vi "AfficherCommande.vi"() -> (0 "Result Set":string[][](table), 1 "Column Names":string[](array[string]))   [LabVIEW 2024]
uses:
  <vilib>/drjdpowell/SQLite Library/SQL Statement/SQL Statement.lvclass/SQL Statement.ctl
  <vilib>/drjdpowell/SQLite Library/SQL Connection/Open (string).vi
  <vilib>/drjdpowell/SQLite Library/SQL Connection/Execute SQL.vi
  <vilib>/drjdpowell/SQLite Library/SQL Statement/Error Message.vi
  <vilib>/drjdpowell/SQLite Library/SQL Connection/Connection.lvclass
  <vilib>/drjdpowell/SQLite Library/SQLite.lvlib
panel:
  # "Liste des commandes"
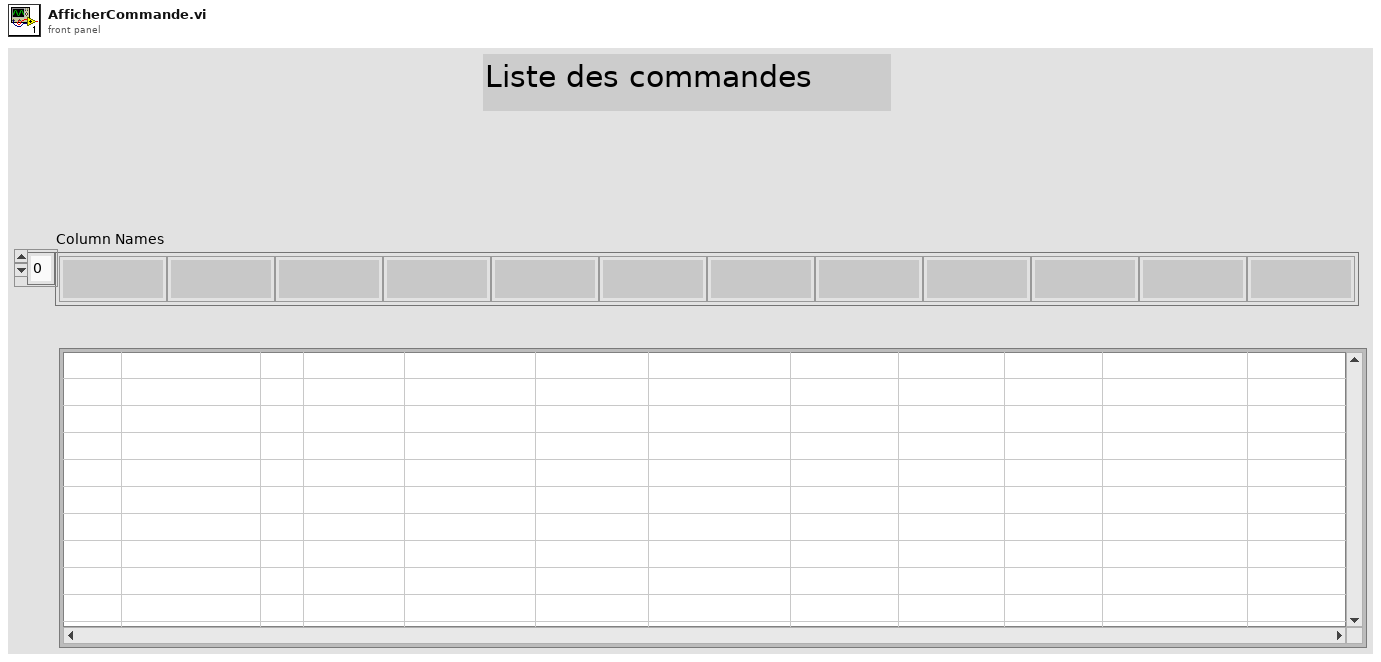
[diagram p1: front panel]
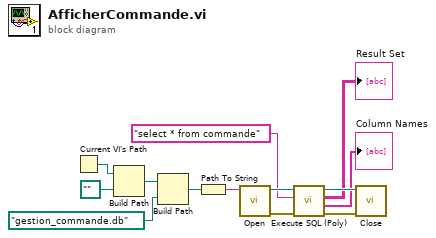
[diagram p0: block diagram]
diagram:
  n1 = Current VI's Path() -> (path=w13:path)
  n2 = Build Path(base path=w13, name or relative path=path "..") -> (appended path=w10:path)
  n3 = Build Path(base path=w10, name or relative path=path "gestion_commande.db" ("Filename")) -> (appended path=w9:path)
  n4 = Path To String(path=w9) -> (string=w1:string)
  n5 = call-poly <vilib>:"Open.vi"("db file"=w1) -> ("error out"=w7:errorcluster, "SQLite Connection"=w8:refnum<class "Connection.lvclass">)  [unwired: 9 in]
  n6 = call-poly <vilib>:"Execute SQL (Poly).vi"("error in (no error)"=w7, "SQL"="select * from commande", "SQLite Connection in"=w8) -> ("error out"=w6:errorcluster, "Column Names"=→"Column Names":string[], "Result Set"=→"Result Set":string[][], "SQLite Connection"=w5:refnum<class "Connection.lvclass">)  [unwired: 5 in]
  n7 = call-dynamic "Close.vi"("error in (no error)"=w6, "SQLite Connection in"=w5) -> ()  [unwired: 9 in, 1 out]
